vi "cm2nm_modify_spot_info.vi"(6 "Is Fiducial":bool, 8 "TransformedPt":bool, 9 "ArrayOfSpotNames":string[](array[string]), 10 "Current Session Information":T1={"CollectionOfPoints"=[{"MetaDataFile"=path "/INL Macintosh/Users/timothymcjunkin/Desktop/Diffusion couple/MXRD 9-13-10/Fid1.UXD", "X"=-4782.0, "Y"=12990.0, "Group"=1, "Z"=350.3, "Rotation"=1.5707963267948966, "Fiducial"=TRUE, "Magnification"=0.0, "Working_Distance"=0.0, "Notes"="", "Location Name/ID"="F1", "OtherRelatedDataFiles"=[], "Available"=TRUE}, {"MetaDataFile"=path "/INL Macintosh/Users/timothymcjunkin/Desktop/Diffusion couple/MXRD 9-13-10/Fid3B.UXD", "X"=-12864.0, "Y"=-4936.0, "Group"=1, "Z"=512.5999999999999, "Rotation"=1.5707963267948966, "Fiducial"=TRUE, "Magnification"=0.0, "Working_Distance"=0.0, "Notes"="", "Location Name/ID"="F3B", "OtherRelatedDataFiles"=[], "Available"=FALSE}, {"MetaDataFile"=path "/INL Macintosh/Users/timothymcjunkin/Desktop/Diffusion couple/MXRD 9-13-10/Fid5C.UXD", "X"=4762.0, "Y"=-13159.0, "Group"=1, "Z"=512.5999999999999, "Rotation"=1.5707963267948966, "Fiducial"=TRUE, "Magnification"=0.0, "Working_Distance"=0.0, "Notes"="", "Location Name/ID"="F5C", "OtherRelatedDataFiles"=[], "Available"=TRUE}, {"MetaDataFile"=path "", "X"=162.40381449303823, "Y"=-31.01324453854977, "Group"=1, "Z"=430.4482310236498, "Rotation"=0.0, "Fiducial"=FALSE, "Magnification"=0.0, "Working_Distance"=0.0, "Notes"="", "Location Name/ID"="Interface_corrected", "OtherRelatedDataFiles"=[], "Available"=FALSE}, {"MetaDataFile"=path "/INL Macintosh/Users/timothymcjunkin/Desktop/Diffusion couple/MXRD 9-13-10/Center.UXD", "X"=163.0, "Y"=44.0, "Group"=1, "Z"=-192.39999999999998, "Rotation"=-0.8089757988093471, "Fiducial"=FALSE, "Magnification"=0.0, "Working_Distance"=0.0, "Notes"="", "Location Name/ID"="interface_Manual_find", "OtherRelatedDataFiles"=[], "Available"=FALSE}, {"MetaDataFile"=path "", "X"=1407.972144786283, "Y"=-1304.0831828104674, "Group"=1, "Z"=435.6245662356068, "Rotation"=0.0, "Fiducial"=FALSE, "Magnification"=0.0, "Working_Distance"=0.0, "Notes"="", "Location Name/ID"="Corner_correcte_S1", "OtherRelatedDataFiles"=[], "Available"=FALSE}, {"MetaDataFile"=path "/INL Macintosh/Users/timothymcjunkin/Desktop/Diffusion couple/MXRD 9-13-10/Corner.UXD", "X"=1397.752237926863, "Y"=-1316.5905644166705, "Group"=1, "Z"=435.75379333055236, "Rotation"=-0.6331076967321386, "Fiducial"=FALSE, "Magnification"=0.0, "Working_Distance"=0.0, "Notes"="", "Location Name/ID"="Corner_correcte_S1_fix", "OtherRelatedDataFiles"=[], "Available"=FALSE}], "Instrument"=3, "CollectionFile"=path "/INL Macintosh/Users/timothymcjunkin/Desktop/Diffusion couple/MXRD 9-13-10/xrd_session_for_corrected.xml", "Session Name/ID"="xrd_test", "SessionNotes"="Sample moved to XRD"} {"Instrument" items=["Unknown", "Phillips SEM IRC", "JEOL 7000F EML_MFC", "MXRD MFC", "JEOL_EPMA"]; "CollectionOfPoints"."Rotation" min=-37480660.29033894 max=37480660.27288565}, 11 "Input of Spot information":T2={"MetaDataFile"=path "/INL Macintosh/Users/timothymcjunkin/Desktop/Diffusion couple/MXRD 9-13-10/Corner.UXD", "X"=1346.0, "Y"=-1254.0, "Group"=0, "Z"=-87.9, "Rotation"=-0.6331076967321386, "Fiducial"=FALSE, "Magnification"=0.0, "Working_Distance"=0.0, "Notes"="", "Location Name/ID"="", "OtherRelatedDataFiles"=[], "Available"=FALSE} {"Rotation" min=-37480660.29033894 max=37480660.27288565}) -> (0 "Output of Spot information":T2={"MetaDataFile"=path "/INL Macintosh/Users/timothymcjunkin/Desktop/Diffusion couple/MXRD 9-13-10/Corner.UXD", "X"=1346.0, "Y"=-1254.0, "Group"=0, "Z"=-87.9, "Rotation"=-0.6331076967321386, "Fiducial"=FALSE, "Magnification"=0.0, "Working_Distance"=0.0, "Notes"="", "Location Name/ID"="", "OtherRelatedDataFiles"=[], "Available"=FALSE} {"Rotation" min=-37480660.29033894 max=37480660.27288565}, 1 "Current Session Information Out":T1={"CollectionOfPoints"=[{"MetaDataFile"=path "/INL Macintosh/Users/timothymcjunkin/Desktop/Diffusion couple/MXRD 9-13-10/Fid1.UXD", "X"=-4782.0, "Y"=12990.0, "Group"=1, "Z"=350.3, "Rotation"=1.5707963267948966, "Fiducial"=TRUE, "Magnification"=0.0, "Working_Distance"=0.0, "Notes"="", "Location Name/ID"="F1", "OtherRelatedDataFiles"=[], "Available"=TRUE}, {"MetaDataFile"=path "/INL Macintosh/Users/timothymcjunkin/Desktop/Diffusion couple/MXRD 9-13-10/Fid3B.UXD", "X"=-12864.0, "Y"=-4936.0, "Group"=1, "Z"=512.5999999999999, "Rotation"=1.5707963267948966, "Fiducial"=TRUE, "Magnification"=0.0, "Working_Distance"=0.0, "Notes"="", "Location Name/ID"="F3B", "OtherRelatedDataFiles"=[], "Available"=FALSE}, {"MetaDataFile"=path "/INL Macintosh/Users/timothymcjunkin/Desktop/Diffusion couple/MXRD 9-13-10/Fid5C.UXD", "X"=4762.0, "Y"=-13159.0, "Group"=1, "Z"=512.5999999999999, "Rotation"=1.5707963267948966, "Fiducial"=TRUE, "Magnification"=0.0, "Working_Distance"=0.0, "Notes"="", "Location Name/ID"="F5C", "OtherRelatedDataFiles"=[], "Available"=TRUE}, {"MetaDataFile"=path "", "X"=162.40381449303823, "Y"=-31.01324453854977, "Group"=1, "Z"=430.4482310236498, "Rotation"=0.0, "Fiducial"=FALSE, "Magnification"=0.0, "Working_Distance"=0.0, "Notes"="", "Location Name/ID"="Interface_corrected", "OtherRelatedDataFiles"=[], "Available"=FALSE}, {"MetaDataFile"=path "/INL Macintosh/Users/timothymcjunkin/Desktop/Diffusion couple/MXRD 9-13-10/Center.UXD", "X"=163.0, "Y"=44.0, "Group"=1, "Z"=-192.39999999999998, "Rotation"=-0.8089757988093471, "Fiducial"=FALSE, "Magnification"=0.0, "Working_Distance"=0.0, "Notes"="", "Location Name/ID"="interface_Manual_find", "OtherRelatedDataFiles"=[], "Available"=FALSE}, {"MetaDataFile"=path "", "X"=1407.972144786283, "Y"=-1304.0831828104674, "Group"=1, "Z"=435.6245662356068, "Rotation"=0.0, "Fiducial"=FALSE, "Magnification"=0.0, "Working_Distance"=0.0, "Notes"="", "Location Name/ID"="Corner_correcte_S1", "OtherRelatedDataFiles"=[], "Available"=FALSE}, {"MetaDataFile"=path "/INL Macintosh/Users/timothymcjunkin/Desktop/Diffusion couple/MXRD 9-13-10/Corner.UXD", "X"=1397.752237926863, "Y"=-1316.5905644166705, "Group"=1, "Z"=435.75379333055236, "Rotation"=-0.6331076967321386, "Fiducial"=FALSE, "Magnification"=0.0, "Working_Distance"=0.0, "Notes"="", "Location Name/ID"="Corner_correcte_S1_fix", "OtherRelatedDataFiles"=[], "Available"=FALSE}], "Instrument"=3, "CollectionFile"=path "/INL Macintosh/Users/timothymcjunkin/Desktop/Diffusion couple/MXRD 9-13-10/xrd_session_for_corrected.xml", "Session Name/ID"="xrd_test", "SessionNotes"="Sample moved to XRD"} {"Instrument" items=["Unknown", "Phillips SEM IRC", "JEOL 7000F EML_MFC", "MXRD MFC", "JEOL_EPMA"]; "CollectionOfPoints"."Rotation" min=-37480660.29033894 max=37480660.27288565}, 3 "Cancel":bool)   [LabVIEW 2010]
uses:
  cm2nm_coordinate_information_v2.ctl
  cm2nm_sample_set.ctl
panel:
  in  "Group Coding":i32
  in  "Boolean 2":bool
  in  "Boolean":bool
  out "MetaDataAvailable":bool caption="Is a Fiducial"
  out "error out":errorcluster
  in  "Is a Fiducial":bool
  in  "Notes:":string
  in  "Tab Control":T3(tab)
  in  "Tilt":dbl
  in  "Stage Rotation":dbl
  in  "Get Coordinates from Meta File":bool
  in  "Press to Move to Next\nInformation Screen":bool
  in  "Spot Name":string
  in  "Z-Position":dbl
  in  "Y-Position":dbl
  in  "X-Position":dbl
  in  "MetaDataFile":path
  in  "Cancel2":bool caption="Cancel Adding \nthis Point to \nthe DataBase"
  in  "Add A Spot Related Data File":bool caption="Add Another File\nRelated to this Spot"
  in  "Goto Previous Screen":bool caption="Press to Move to \nPrevious Screen"
  in  "Press to goto final Screen":bool caption="Press to Move to Next\nInformation Screen"
  out "OtherRelatedDataFiles":T4(array[cluster])
  in  "Cancel3":bool caption="Cancel Adding \nthis Point to \nthe DataBase"
  in  "Go Back to Correct":bool caption="Some information\nis Incorrect or \nWrong"
  in  "Cancel":bool caption="Cancel Adding \nthis Point to \nthe DataBase"
  in  "AddToDataBase":bool caption="Information is\nCorrect Add the\nPoint"
  # "Enter or confirm the\nspot  name and positions\n\nIf Metafile is available \nselect it in the MetaDatafile\nField and click Use MetaFile\nto extract MetaData\nFrom the file."
  # "This form allows you\nto add any number of\nfiles related to this\nspot on the sample.\nFor example spectra\nfiles or images other\nthan the file \ncontaining meta data."
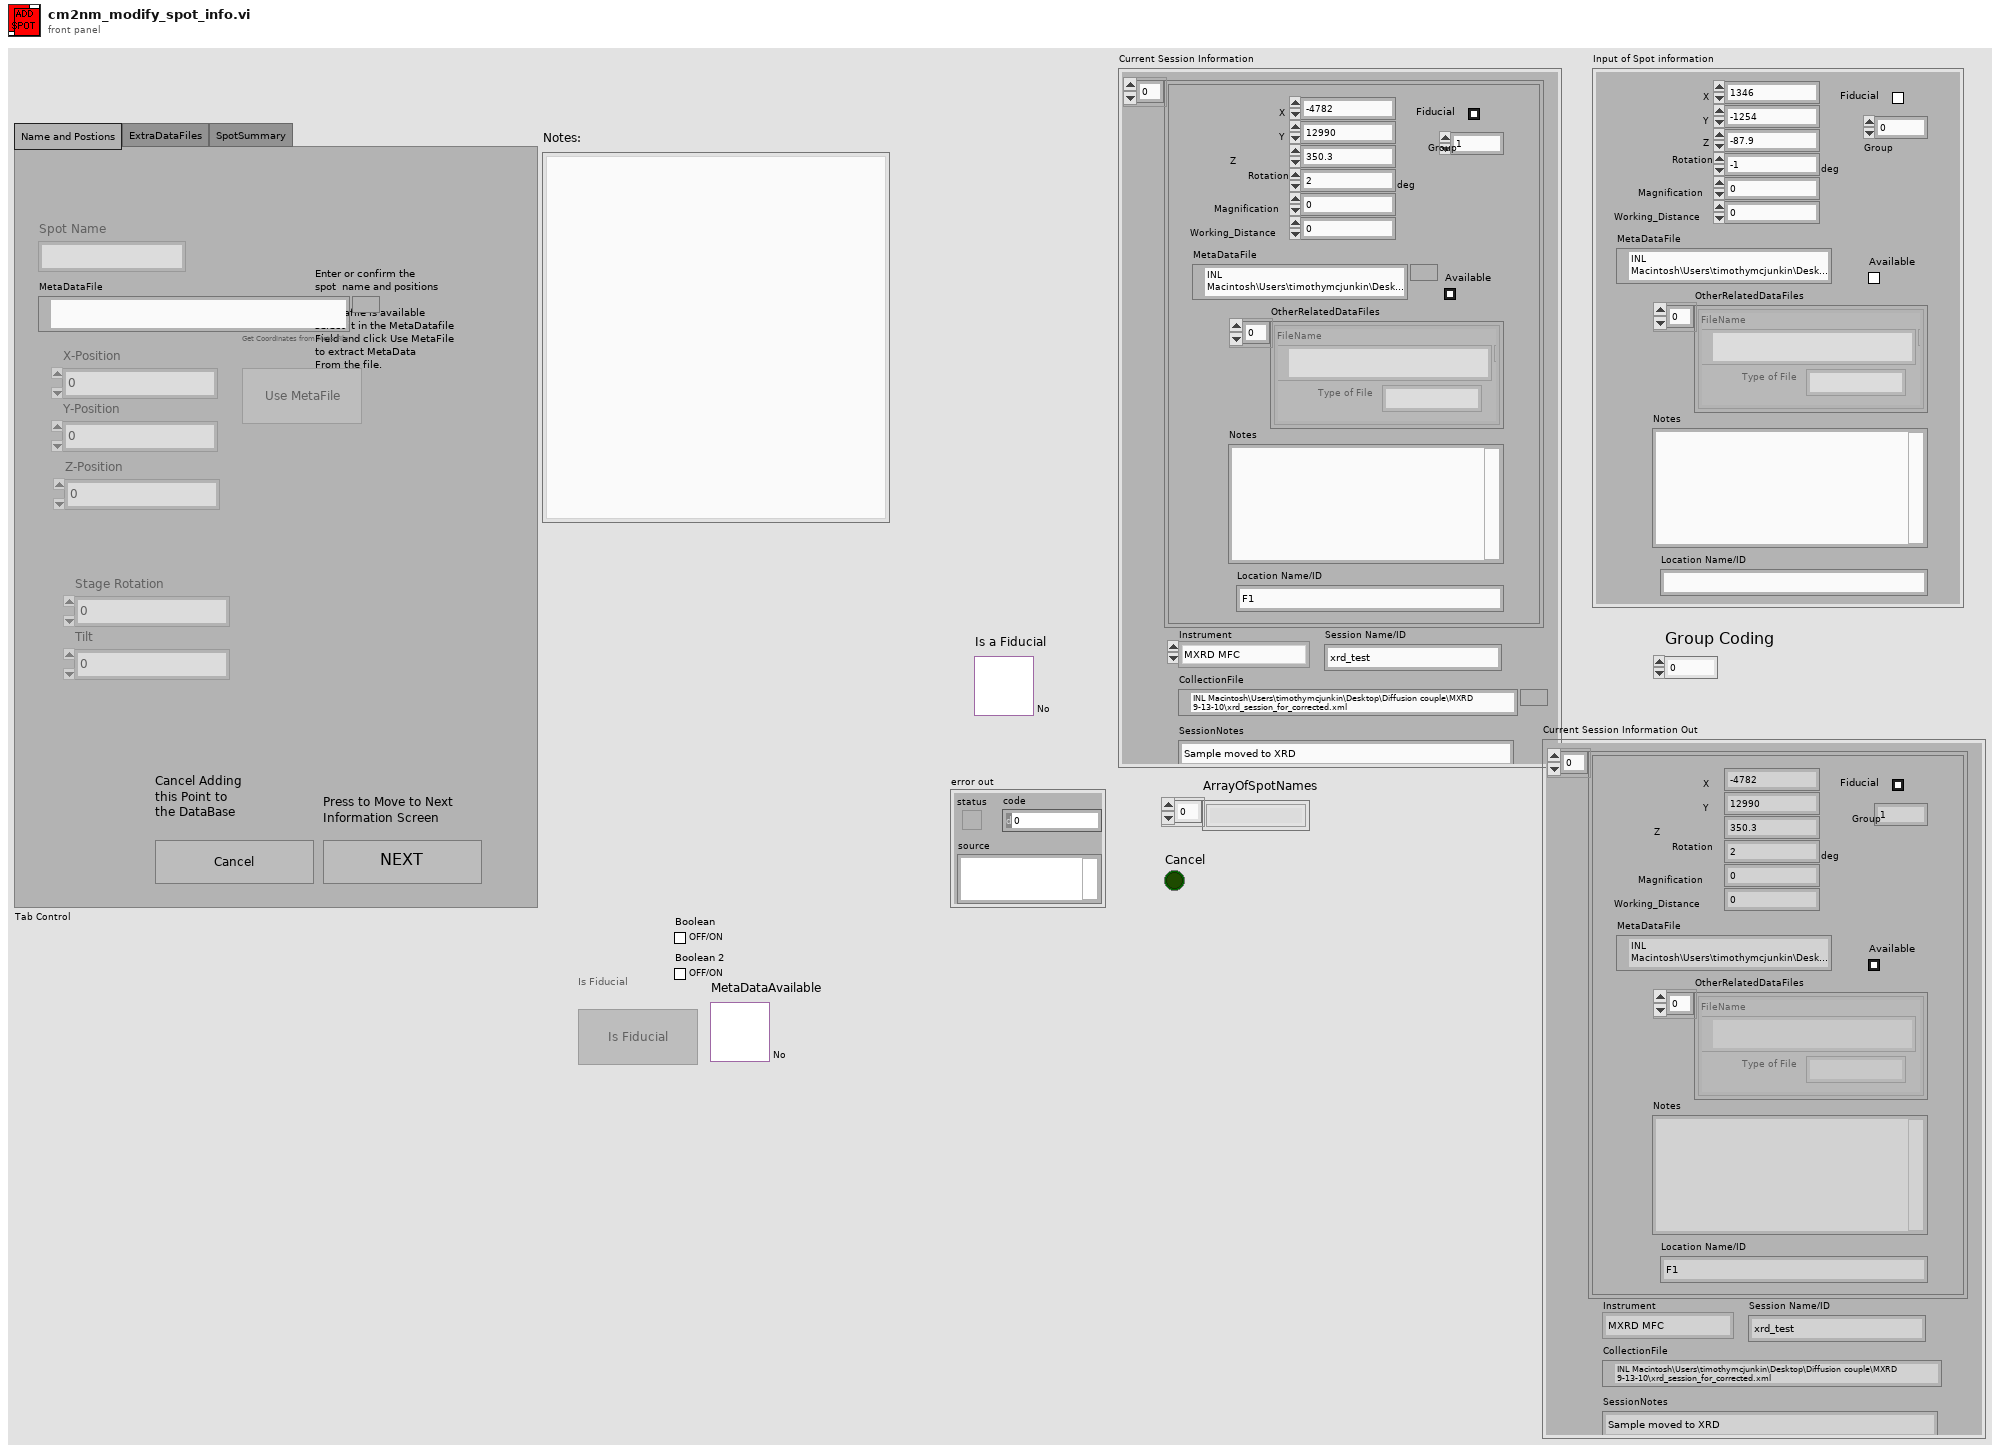
[diagram p1: front panel]
types:
  T1 = typedef "cm2nm_sample_set.ctl" = cluster{"CollectionOfPoints":T2[], "Instrument":u16, "CollectionFile":path, "Session Name/ID":string, "SessionNotes":string}
  T2 = typedef "cm2nm_coordinate_information_v2.ctl" = cluster{"MetaDataFile":path, "X":dbl, "Y":dbl, "Group":i32, "Z":dbl, "Rotation":dbl[unit], "Fiducial":bool, "Magnification":dbl, "Working_Distance":dbl, "Notes":string, "Location Name/ID":string, "OtherRelatedDataFiles":cluster{"Type of File":string, "FileName":path}[], "Available":bool}
  T3 = enum32{"Name and Postions", "ExtraDataFiles", "SpotSummary"}
  T4 = cluster{"Type of File":string, "FileName":path}[]
  T5 = enum32{"Name and Postions", "ExtraDataFiles", "SpotSummary", "Inputs"}
  T6 = enum8{"Enabled", "Disabled", "Disabled and Grayed Out"}
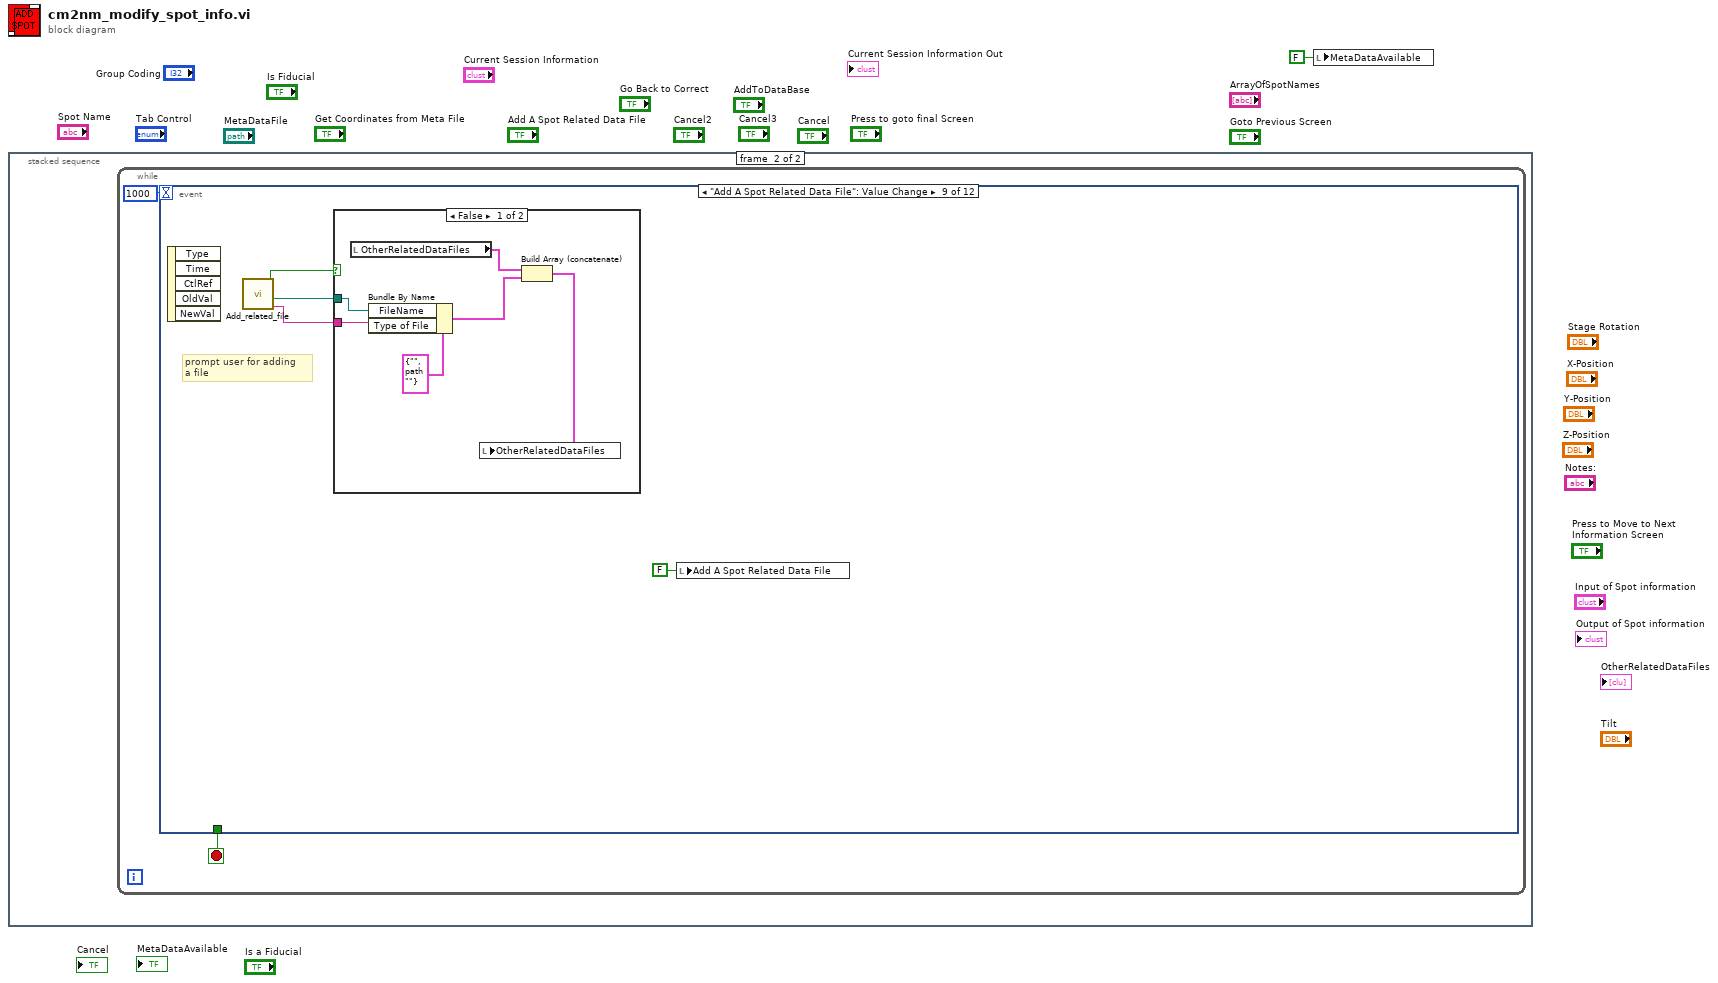
[diagram p0: block diagram]
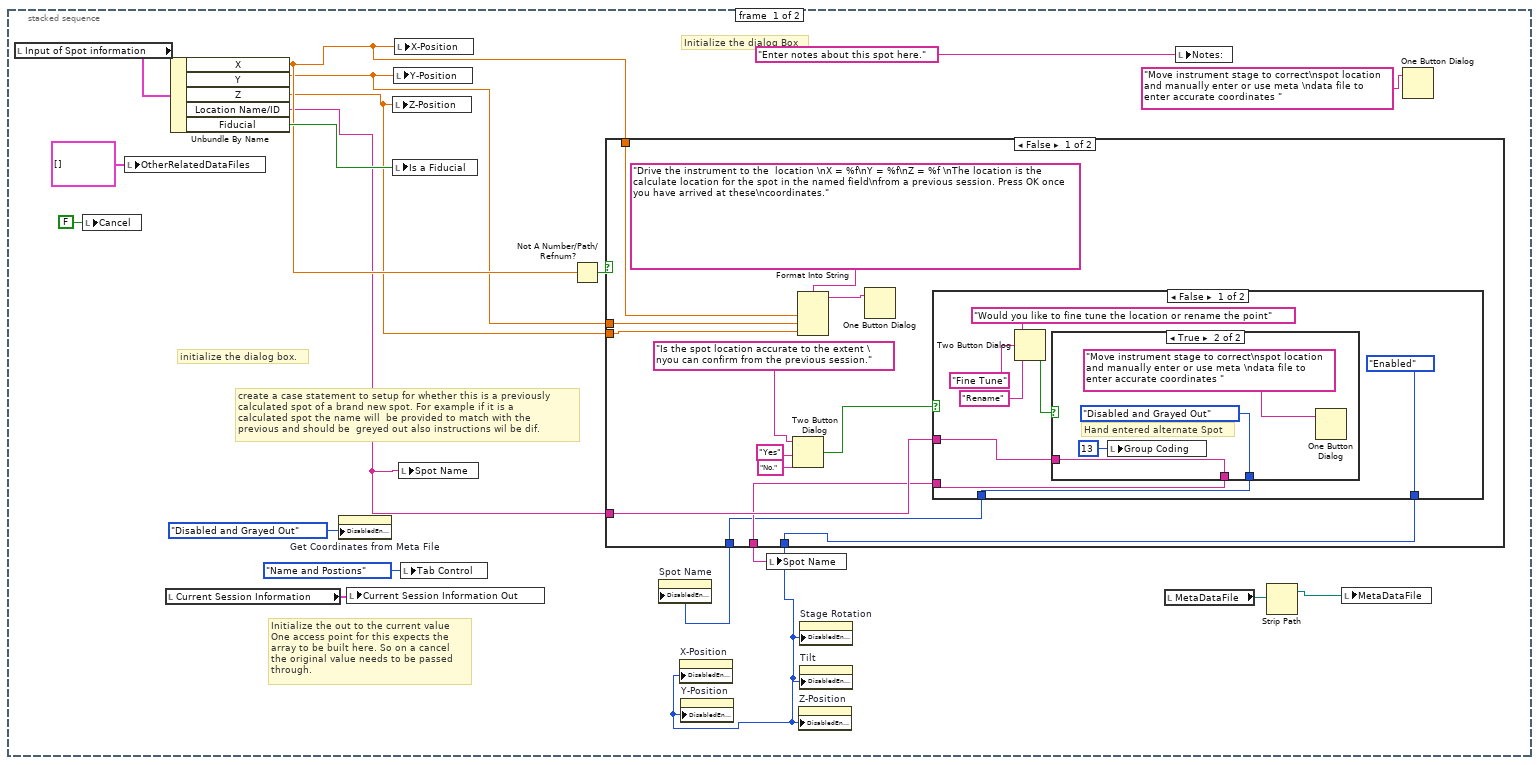
[diagram p2: hidden frame]
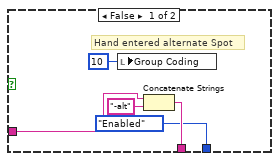
[diagram p3: hidden frame]
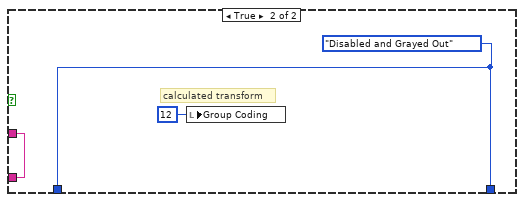
[diagram p4: hidden frame]
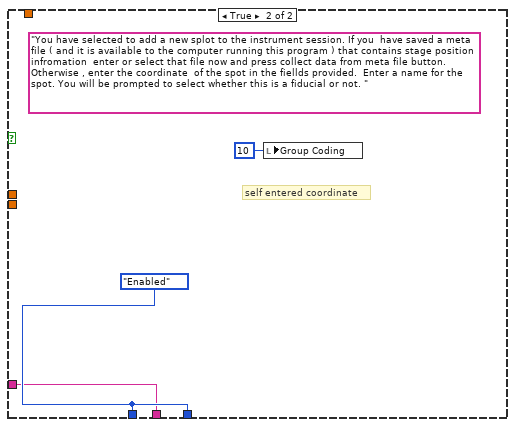
[diagram p5: hidden frame]
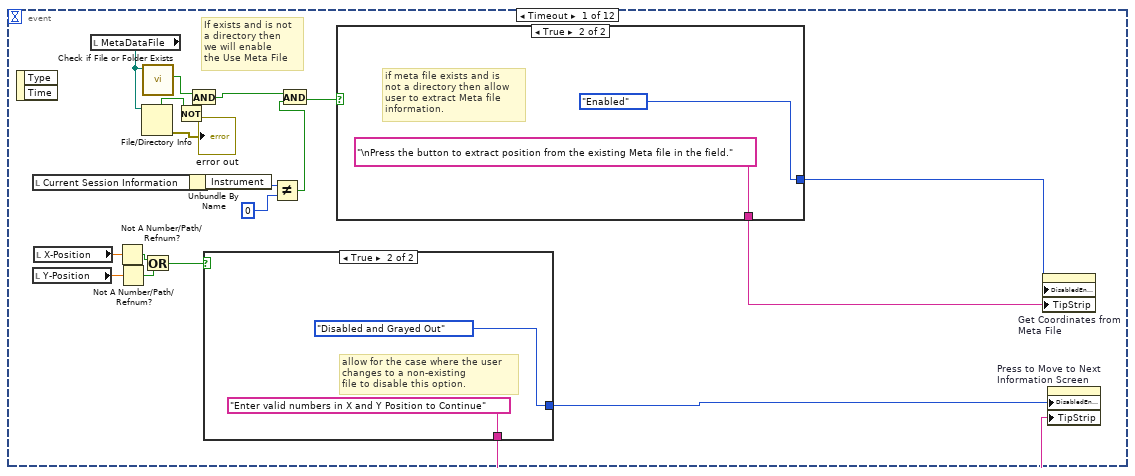
[diagram p6: hidden frame]
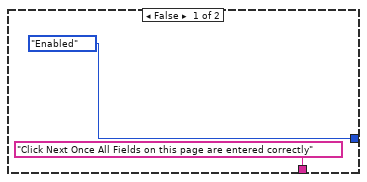
[diagram p7: hidden frame]
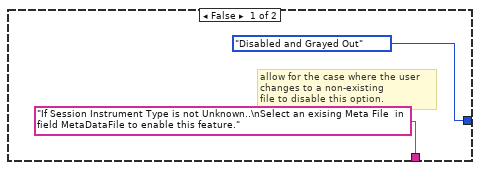
[diagram p8: hidden frame]
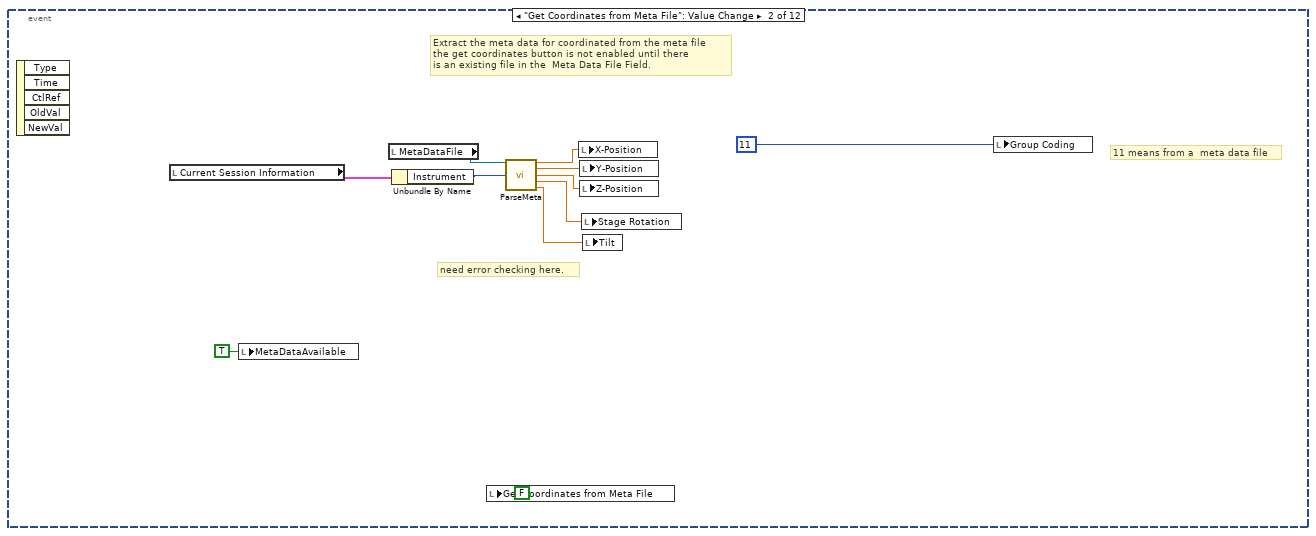
[diagram p9: hidden frame]
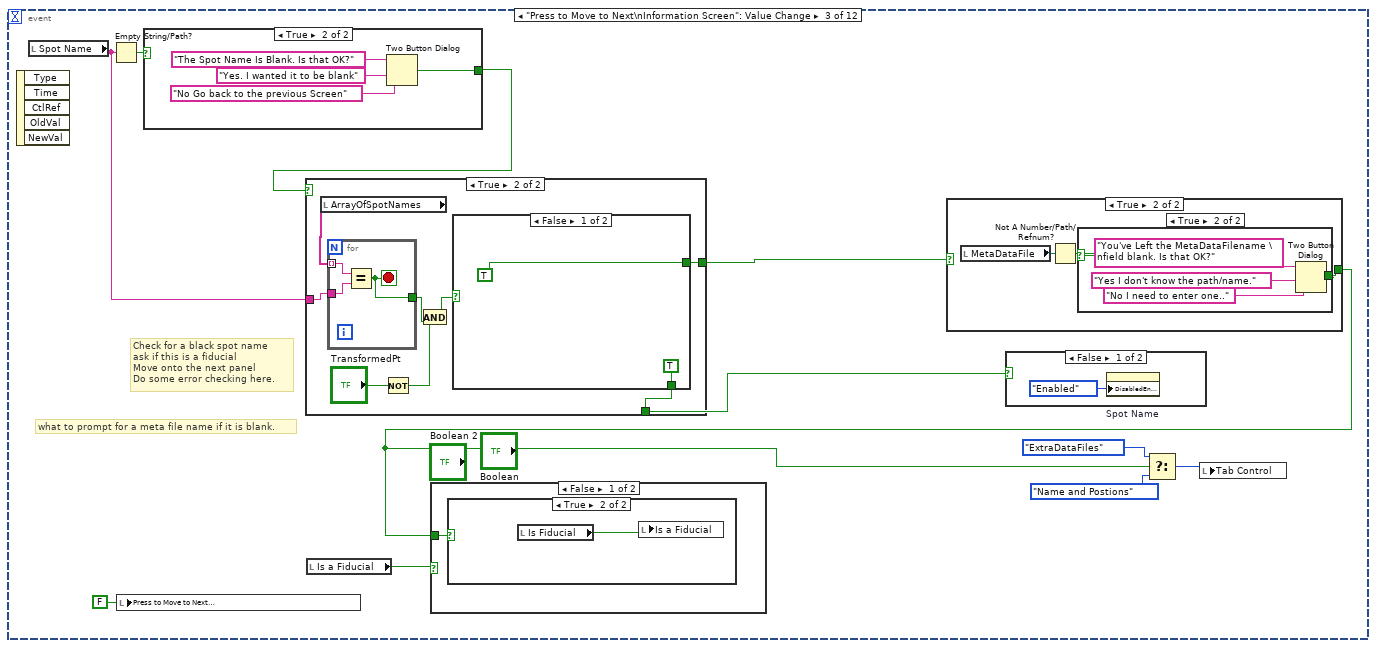
[diagram p10: hidden frame]
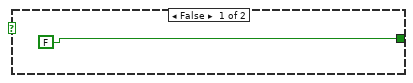
[diagram p14: hidden frame]
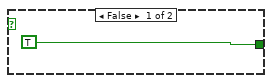
[diagram p15: hidden frame]
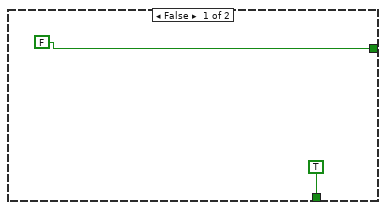
[diagram p16: hidden frame]
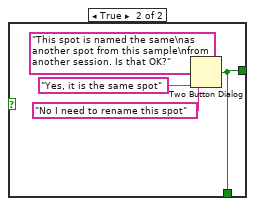
[diagram p17: hidden frame]
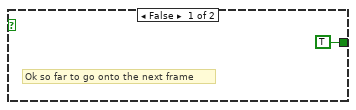
[diagram p18: hidden frame]
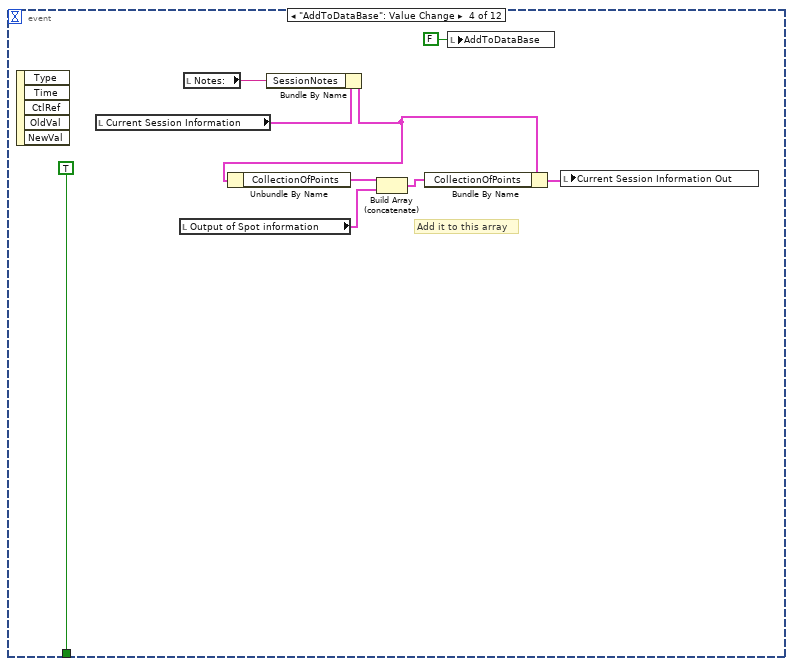
[diagram p19: hidden frame]
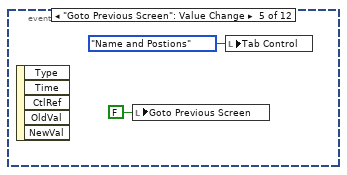
[diagram p20: hidden frame]
diagram:
  n1 = stacked-sequence {
    frame #0 {
      # "Initialize the out to the current value\nOne access point for this expects the\narray to be built here. So on a cancel\nthe original value needs to be passed\nthrough."
      # "Initialize the dialog Box"
      # "create a case statement to setup for whether this is a previously\ncalculated spot of a brand new spot. For example if it is a\ncalculated spot the name will  be provided to match with the \nprevious and should be  greyed out also instructions wil be dif."
      # "initialize the dialog box."
      n2 = local read "Input of Spot information"() -> (w20:T2)
      n3 = local write "Cancel"(FALSE ("Cancel")) -> ()
      n4 = local write "OtherRelatedDataFiles"(T4 [] ("OtherRelatedDataFiles")) -> ()
      n5 = local read "Current Session Information"() -> (w8:T1)
      n6 = Unbundle By Name(w20) -> ("X"=w16:dbl, "Y"=w15:dbl, "Z"=w3:dbl, "Location Name/ID"=w6:string, "Fiducial"=w19:bool)
      n7 = property on="Get Coordinates from Meta File" class="Bool (strict)"("DisabledEnum"=T6."Disabled and Grayed Out" ("Disabled")) -> ()  [unwired: 2 in, 2 out]
      n8 = local write "Current Session Information Out"(w8) -> ()
      n9 = local write "Z-Position"(w3) -> ()
      n10 = local write "Is a Fiducial"(w19) -> ()
      n11 = local write "Y-Position"(w15) -> ()
      n12 = local write "X-Position"(w16) -> ()
      n13 = local write "Spot Name"(w6) -> ()
      n14 = local write "Tab Control"(T5."Name and Postions" ("Tab Control")) -> ()
      n15 = Not A Number/Path/Refnum?(number/path/refnum=w16) -> (NaN/Path/Refnum?=w18:bool)
      n16 = case shown="False" w18 {
        tunnel: [w24 w56] -> w14
        tunnel: w16 -> [w32 _]
        tunnel: w15 -> [w31 _]
        tunnel: [w21 w56] -> w13
        tunnel: w6 -> [w23 w55]
        tunnel: [w22 w55] -> w12
        tunnel: w3 -> [w26 _]
        frame False {
          n17 = Two Button Dialog(message="Is the spot location accurate to the extent \nyou can confirm from the previous session.", 1:"No." ("F button name (\"Cancel\")"), 2:"Yes" ("T button name (\"OK\")")) -> (T button?=w25:bool)
          n18 = Format Into String(format string="Drive the instrument to the  location \nX = %f\nY = %f\nZ = %f \nThe location is the calculate location for the spot in the named field\nfrom a previous session. Press OK once you have arrived at these\ncoordinates.", w32, w31, w26) -> (resulting string=w30:string)  [unwired: 2 in, 1 out]
          n19 = One Button Dialog ("Drive to the Calculated Coordinates")(message=w30) -> ()  [unwired: 1 in, 1 out]
          n20 = case shown="False" w25 {
            tunnel: [T6."Enabled" ("Disabled") w52] -> w24
            tunnel: w23 -> [w36 w53]
            tunnel: [w35 w53] -> w22
            tunnel: [w34 w52] -> w21
            frame False {
              n21 = Two Button Dialog(message="Would you like to fine tune the location or rename the point", 1:"Rename" ("F button name (\"Cancel\")"), 2:"Fine Tune" ("T button name (\"OK\")")) -> (T button?=w37:bool)
              n22 = case shown="True" w37 {
                tunnel: w36 -> [w45 w50]
                tunnel: [w44 w50] -> w35
                tunnel: [T6."Enabled" ("Disabled") T6."Disabled and Grayed Out" ("Disabled")] -> w34
                frame False {
                  # "Hand entered alternate Spot"
                  n23 = local write "Group Coding"(10 ("Group Coding")) -> ()
                  n24 = Concatenate Strings(w45, "-alt" ("string")) -> (w44:string)
                }
                frame True {
                  # "Hand entered alternate Spot"
                  n25 = local write "Group Coding"(13 ("Group Coding")) -> ()
                  n26 = One Button Dialog ("Drive to the Calculated Coordinates")(message="Move instrument stage to correct\nspot location and manually enter or use meta \ndata file to enter accurate coordinates ") -> ()  [unwired: 1 in, 1 out]
                }
              }
            }
            frame True {
              w52 = T6."Disabled and Grayed Out" ("Disabled")
              # "calculated transform"
              n27 = local write "Group Coding"(12 ("Group Coding")) -> ()
            }
          }
        }
        frame True {
          w56 = T6."Enabled" ("Disabled")
          (unwired) "You have selected to add a new splot to the instrument session. If you  have saved a meta file ( and it is available to the computer running this program ) that contains stage position infromation  enter or select that file now and press collect data from meta file button. Otherwise , enter the coordinate  of the spot in the fiellds provided.  Enter a name for the spot. You will be prompted to select whether this is a fiducial or not. "
          # "self entered coordinate"
          n28 = local write "Group Coding"(10 ("Group Coding")) -> ()
        }
      }
      n29 = property on="Spot Name" class="Str"("DisabledEnum"=w13) -> ()  [unwired: 2 in, 2 out]
      n30 = property on="X-Position" class="DigNum (strict)"("DisabledEnum"=w14) -> ()  [unwired: 2 in, 2 out]
      n31 = property on="Y-Position" class="DigNum (strict)"("DisabledEnum"=w14) -> ()  [unwired: 2 in, 2 out]
      n32 = local write "Spot Name"(w12) -> ()
      n33 = property on="Z-Position" class="DigNum (strict)"("DisabledEnum"=w14) -> ()  [unwired: 2 in, 2 out]
      n34 = property on="Stage Rotation" class="DigNum (strict)"("DisabledEnum"=w14) -> ()  [unwired: 2 in, 2 out]
      n35 = property on="Tilt" class="DigNum (strict)"("DisabledEnum"=w14) -> ()  [unwired: 2 in, 2 out]
      n36 = local read "MetaDataFile"() -> (w5:path)
      n37 = local write "Notes:"("Enter notes about this spot here." ("Notes:")) -> ()
      n38 = Strip Path(path=w5) -> (stripped path=w4:path)  [unwired: 1 out]
      n39 = local write "MetaDataFile"(w4) -> ()
      n40 = One Button Dialog ("Drive to the Calculated Coordinates")(message="Move instrument stage to correct\nspot location and manually enter or use meta \ndata file to enter accurate coordinates ") -> ()  [unwired: 1 in, 1 out]
    }
    frame #1 {
      n41 = while {
        stop <- w57 stop-if-true
        n42 = event shown="[8] \"Add A Spot Related Data File\": Value Change" {
          selector: _ -> [_ _ _ _ _ _ _ _ _ _ _ _]
          dyn-events: _ -> [_ _ _ _ _ _ _ _ _ _ _ _]
          timeout: 1000 -> [_ _ _ _ _ _ _ _ _ _ _ _]
          tunnel: [_ _ _ TRUE ("T button?") _ _ _ w188 _ _ _ _] -> w57
          event Timeout {
            # "If exists and is not\na directory then\nwe will enable \nthe Use Meta File"
            n43 = event-data() -> ()  [unwired: 1 in, 2 out]
            n44 = local read "Current Session Information"() -> (w63:T1)
            n45 = local read "Y-Position"() -> (w67:dbl)
            n46 = local read "X-Position"() -> (w68:dbl)
            n47 = local read "MetaDataFile"() -> (w71:path)
            n48 = Not A Number/Path/Refnum?(number/path/refnum=w68) -> (NaN/Path/Refnum?=w66:bool)
            n49 = Not A Number/Path/Refnum?(number/path/refnum=w67) -> (NaN/Path/Refnum?=w65:bool)
            n50 = File/Directory Info(path=w71) -> (directory=w78:bool, error out=→"error out":errorcluster)  [unwired: 1 in, 5 out]
            n51 = call <vilib>:"Check if File or Folder Exists.vi"("path"=w71) -> ("file or folder exists?"=w76:bool)  [unwired: 8 in, 2 out]
            n52 = Or(x=w66, y=w65) -> (x .or. y?=w64:bool)
            n53 = Not(x=w78) -> (.not. x?=w77:bool)
            n54 = And(x=w76, y=w77) -> (x .and. y?=w72:bool)
            n55 = Unbundle By Name(w63) -> ("Instrument"=w62:u16)
            n56 = case shown="True" w64 {
              tunnel: [T6."Enabled" ("Disabled") T6."Disabled and Grayed Out" ("Disabled")] -> w70
              tunnel: ["Click Next Once All Fields on this page are entered correctly" ("Tip Strip") "Enter valid numbers in X and Y Position to Continue" ("Tip Strip")] -> w69
              frame False {
              }
              frame True {
                # "allow for the case where the user\nchanges to a non-existing\nfile to disable this option."
              }
            }
            n57 = Not Equal?(x=w62, y=u16 0) -> (x != y?=w59:bool)
            n58 = And(x=w72, y=w59) -> (x .and. y?=w60:bool)
            n59 = case shown="True" w60 {
              tunnel: [T6."Disabled and Grayed Out" ("Disabled") T6."Enabled" ("Disabled")] -> w74
              tunnel: ["If Session Instrument Type is not Unknown..\nSelect an exising Meta File  in field MetaDataFile to enable this feature." ("Tip Strip") "\nPress the button to extract position from the existing Meta file in the field." ("Tip Strip")] -> w73
              frame False {
                # "allow for the case where the user\nchanges to a non-existing\nfile to disable this option."
              }
              frame True {
                # "if meta file exists and is\nnot a directory then allow \nuser to extract Meta file \ninformation."
              }
            }
            n60 = property on="Get Coordinates from Meta File" class="Bool (strict)"("DisabledEnum"=w74, "TipStrip"=w73) -> ()  [unwired: 2 in, 2 out]
            n61 = property on="Press to Move to Next\nInformation Screen" class="Bool (strict)"("DisabledEnum"=w70, "TipStrip"=w69) -> ()  [unwired: 2 in, 2 out]
          }
          event "Get Coordinates from Meta File": Value Change {
            # "11 means from a  meta data file"
            # "need error checking here."
            # "Extract the meta data for coordinated from the meta file\nthe get coordinates button is not enabled until there\nis an existing file in the  Meta Data File Field."
            n62 = event-data() -> ()  [unwired: 1 in, 5 out]
            n63 = local read "Current Session Information"() -> (w88:T1)
            n64 = local write "MetaDataAvailable"(TRUE ("MetaDataAvailable")) -> ()
            n65 = local read "MetaDataFile"() -> (w96:path)
            n66 = Unbundle By Name(w88) -> ("Instrument"=w95:u16)
            n67 = local write "Get Coordinates from Meta File"(FALSE ("Get Coords")) -> ()
            n68 = call "ParseMeta.vi"("Path"=w96, "Instrument"=w95) -> ("X-stage (um)"=w94:dbl, "Y-stage (um)"=w93:dbl, "Z-stage (um)"=w92:dbl, "R-stage (deg)"=w91:dbl, "StageTilt"=w90:dbl)  [unwired: 1 in, 8 out]
            n69 = local write "X-Position"(w94) -> ()
            n70 = local write "Y-Position"(w93) -> ()
            n71 = local write "Z-Position"(w92) -> ()
            n72 = local write "Stage Rotation"(w91) -> ()
            n73 = local write "Tilt"(w90) -> ()
            n74 = local write "Group Coding"(11 ("Group Coding")) -> ()
          }
          event "Press to Move to Next\nInformation Screen": Value Change {
            # "what to prompt for a meta file name if it is blank."
            # "Check for a black spot name\nask if this is a fiducial\nMove onto the next panel\nDo some error checking here."
            n75 = event-data() -> ()  [unwired: 1 in, 5 out]
            n76 = local read "Spot Name"() -> (w105:string)
            n77 = Empty String/Path?(string/path=w105) -> (empty?=w107:bool)
            n78 = local write "Press to Move to Next\nInformation Screen"(FALSE ("Press to Move to Next\nInformation Screen")) -> ()
            n79 = case shown="True" w107 {
              tunnel: [TRUE ("T button?") w141] -> w106
              frame False {
                # "Ok so far to go onto the next frame"
              }
              frame True {
                n80 = Two Button Dialog(message="The Spot Name Is Blank. Is that OK?", 1:"No Go back to the previous Screen" ("F button name (\"Cancel\")"), 2:"Yes. I wanted it to be blank" ("T button name (\"OK\")")) -> (T button?=w141:bool)
              }
            }
            n81 = case shown="True" w106 {
              tunnel: w105 -> [_ w129]
              tunnel: [FALSE ("T button?") w127] -> w104
              tunnel: [TRUE ("T button?") w126] -> w99
              frame False {
              }
              frame True {
                n82 = local read "ArrayOfSpotNames"() -> (w130:string[])
                n83 = for {
                  tunnel: w130 -> [w139] mode=indexing
                  tunnel: w129 -> [w138]
                  tunnel: [w137] -> w128
                  stop <- w137 stop-if-true
                  n84 = Equal?(x=w139, y=w138) -> (x = y?=w137:bool)
                }
                n85 = Not(x="TransformedPt") -> (.not. x?=w123:bool)
                n86 = And(x=w123, y=w128) -> (x .and. y?=w125:bool)
                n87 = case shown="False" w125 {
                  tunnel: [TRUE ("T button?") w133] -> w127
                  tunnel: [TRUE ("T button?") w133] -> w126
                  frame False {
                  }
                  frame True {
                    n88 = Two Button Dialog(message="This spot is named the same\nas another spot from this sample\nfrom another session. Is that OK?", 1:"No I need to rename this spot" ("F button name (\"Cancel\")"), 2:"Yes, it is the same spot" ("T button name (\"OK\")")) -> (T button?=w133:bool)
                  }
                }
              }
            }
            n89 = local read "Is a Fiducial"() -> (w98:bool)
            n90 = case shown="True" w104 {
              tunnel: [FALSE ("T button?") w113] -> w100
              frame False {
              }
              frame True {
                n91 = local read "MetaDataFile"() -> (w115:path)
                n92 = Not A Number/Path/Refnum?(number/path/refnum=w115) -> (NaN/Path/Refnum?=w114:bool)
                n93 = case shown="True" w114 {
                  tunnel: [TRUE ("T button?") w117] -> w113
                  frame False {
                  }
                  frame True {
                    n94 = Two Button Dialog(message="You've Left the MetaDataFilename \nfield blank. Is that OK?", 1:"No I need to enter one.." ("F button name (\"Cancel\")"), 2:"Yes I don't know the path/name." ("T button name (\"OK\")")) -> (T button?=w117:bool)
                  }
                }
              }
            }
            n95 = case shown="False" w98 {
              tunnel: w100 -> [w109 _]
              frame False {
                n96 = case shown="True" w109 {
                  frame False {
                  }
                  frame True {
                    n97 = local read "Is Fiducial"() -> (w110:bool)
                    n98 = local write "Is a Fiducial"(w110) -> ()
                  }
                }
              }
              frame True {
              }
            }
            n99 = case shown="False" w99 {
              frame False {
                n100 = property on="Spot Name" class="Str"("DisabledEnum"=T6."Enabled" ("Disabled")) -> ()  [unwired: 2 in, 2 out]
              }
              frame True {
              }
            }
            n101 = Select(t=T5."ExtraDataFiles" ("Tab Control"), s=w100, f=T5."Name and Postions" ("Tab Control")) -> (s? t:f=w103:T5)
            n102 = local write "Tab Control"(w103) -> ()
          }
          event "AddToDataBase": Value Change {
            # "Add it to this array"
            n103 = event-data() -> ()  [unwired: 1 in, 5 out]
            n104 = local read "Current Session Information"() -> (w150:T1)
            n105 = local read "Output of Spot information"() -> (w148:T2)
            n106 = local read "Notes:"() -> (w145:string)
            n107 = Bundle By Name(cluster=w150, "SessionNotes"=w145) -> (w146:T1)
            n108 = Unbundle By Name(w146) -> ("CollectionOfPoints"=w149:T2[])
            n109 = Build Array (concatenate)(w149, w148) -> (w147:T2[])
            n110 = Bundle By Name(cluster=w146, "CollectionOfPoints"=w147) -> (w151:T1)
            n111 = local write "AddToDataBase"(FALSE ("AddToDataBase")) -> ()
            n112 = local write "Current Session Information Out"(w151) -> ()
          }
          event "Goto Previous Screen": Value Change {
            n113 = event-data() -> ()  [unwired: 1 in, 5 out]
            n114 = local write "Goto Previous Screen"(FALSE ("Goto Previous Screen")) -> ()
            n115 = local write "Tab Control"(T5."Name and Postions" ("Tab Control")) -> ()
          }
          event "X-Position", "Y-Position", "Z-Position", "MetaDataFile": Value Change {
            # "If user changes any of these from the interface then the values did not come\nfrom the meta file and the indicator should be false."
            n116 = event-data() -> ("CtlRef"=w156:refnum<vi>, "OldVal"=w158:variant, "NewVal"=w157:variant)  [unwired: 1 in, 2 out]
            n117 = local read "Group Coding"() -> (w159:i32)
            n118 = case shown="11" w159 {
              tunnel: w158 -> [_ _ w160]
              tunnel: w157 -> [_ _ _]
              tunnel: w156 -> [_ _ w161]
              frame 0, Default {
              }
              frame 10 {
                # "10 is ok  self entered no warning message for entering these values."
              }
              frame 11 {
                # "coding from meta data file"
                n119 = Two Button Dialog(message="You have modified values\nread from the meta data\nfile or the meta data file name\n. Do you want to do \nthis?  ", 1:"No revert to the old meta data Value" ("F button name (\"Cancel\")"), 2:"Yes, keep the new values" ("T button name (\"OK\")")) -> (T button?=w162:bool)
                n120 = case shown="False" w162 {
                  tunnel: w161 -> [w168 _]
                  tunnel: w160 -> [w166 _]
                  frame False {
                    n121 = property class="Ctl" props=["Value"](reference=w168) -> (reference out=w167:refnum<vi>)  [unwired: 1 in, 2 out]
                    n122 = property class="Ctl"(reference=w167, "Value"=w166) -> ()  [unwired: 1 in, 2 out]
                  }
                  frame True {
                    # "change to 10 so the user\ncan modify as needed"
                    n123 = local write "Group Coding"(10 ("Group Coding")) -> ()
                  }
                }
              }
            }
          }
          event "Spot Name": Value Change {
            n124 = event-data() -> ()  [unwired: 1 in, 5 out]
            n125 = local read "Spot Name"() -> (w170:string)
            n126 = local read "Current Session Information"() -> (w173:T1)
            n127 = Unbundle By Name(w173) -> ("CollectionOfPoints"=w172:T2[])
            n128 = for {
              tunnel: w172 -> [w186] mode=indexing
              tunnel: w170 -> [w184]
              tunnel: [w183] -> w171
              stop <- w183 stop-if-true
              n129 = Unbundle By Name(w186) -> ("Location Name/ID"=w185:string)
              n130 = Equal?(x=w184, y=w185) -> (x = y?=w183:bool)
            }
            n131 = case shown="True" w171 {
              tunnel: w170 -> [_ w179]
              frame False {
              }
              frame True {
                n132 = Random Number (0-1)() -> (number: 0 to 1=w182:dbl)
                n133 = Multiply(x=w182, y=10000) -> (x*y=w177:dbl)
                n134 = Round Toward -Infinity(1:w177) -> (0:w176:dbl)
                n135 = To Unsigned Long Integer(number=w176) -> (unsigned 32bit integer=w175:u32)
                n136 = Format Into String(w175) -> (resulting string=w178:string)  [unwired: 3 in, 1 out]
                n137 = Concatenate Strings(w179, w178) -> (w180:string)
                n138 = property on="Spot Name" class="Str"("Val(Sgnl)"=w180) -> ()  [unwired: 2 in, 2 out]
                n139 = One Button Dialog(message="You have chosen a spot name that duplicates one in this session. \nA random number has been appended to it.") -> ()  [unwired: 1 in, 1 out]
              }
            }
          }
          event "Cancel2", "Cancel3", "Cancel": Value Change {
            w187 = FALSE ("Cancel")
            n140 = event-data() -> ()  [unwired: 1 in, 5 out]
            n141 = Two Button Dialog(message="You have selected cancel adding this spot to the DataBase. Press \"Yes\" if that's what you intended.", 1:"Don't Cancel this Spot" ("F button name (\"Cancel\")"), 2:"YES. do not save this spot" ("T button name (\"OK\")")) -> (T button?=w188:bool)
            n142 = local write "Cancel2"(w187) -> ()
            n143 = local write "Cancel"(w187) -> ()
            n144 = local write "Cancel3"(w187) -> ()
            n145 = local write "Cancel"(w188) -> ()
          }
          event "Add A Spot Related Data File": Value Change {
            # "prompt user for adding\na file"
            n146 = event-data() -> ()  [unwired: 1 in, 5 out]
            n147 = call "Add_related_file.vi"() -> ("Type or Description of File Out"=w193:string, "Path_out"=w194:path, "Cancelled?"=w195:bool)  [unwired: 9 in]
            n148 = case shown="False" w195 {
              tunnel: w194 -> [w199 _]
              tunnel: w193 -> [w198 _]
              frame False {
                n149 = local read "OtherRelatedDataFiles"() -> (w201:T4)
                n150 = Bundle By Name(cluster=cluster{"Type of File":string, "FileName":path} {"Type of File"="", "FileName"=path ""} ("element"), "FileName"=w199, "Type of File"=w198) -> (w197:cluster{"Type of File":string, "FileName":path})
                n151 = Build Array (concatenate)(w201, w197) -> (w196:T4)
                n152 = local write "OtherRelatedDataFiles"(w196) -> ()
              }
              frame True {
              }
            }
            n153 = local write "Add A Spot Related Data File"(FALSE ("Add A Spot Related Data File")) -> ()
          }
          event "Press to goto final Screen": Value Change {
            w203 = 0.0 ("Magnification")
            # "new coding on group\n10 - is a user entered item"
            n154 = event-data() -> ()  [unwired: 1 in, 5 out]
            n155 = local read "Group Coding"() -> (w202:i32)
            n156 = local write "Tab Control"(T3."SpotSummary" ("Tab Control")) -> ()
            n157 = local read "Stage Rotation"() -> (w210:dbl)
            n158 = local read "Is a Fiducial"() -> (w208:bool)
            n159 = local read "Spot Name"() -> (w205:string)
            n160 = local read "MetaDataFile"() -> (w214:path)
            n161 = local read "OtherRelatedDataFiles"() -> (w204:T4)
            n162 = local write "Press to goto final Screen"(FALSE ("Press to goto final Screen")) -> ()
            n163 = local read "Z-Position"() -> (w211:dbl)
            n164 = local read "X-Position"() -> (w212:dbl)
            n165 = local read "Y-Position"() -> (w213:dbl)
            n166 = local read "MetaDataAvailable"() -> (w207:bool)
            n167 = local read "Notes:"() -> (w206:string)
            n168 = node(w210) -> (w209:dbl[unit])
            n169 = Bundle By Name(cluster=T2 {"MetaDataFile"=path "", "X"=nan, "Y"=nan, "Group"=0, "Z"=0.0, "Rotation"=0.0, "Fiducial"=FALSE, "Magnification"=0.0, "Working_Distance"=0.0, "Notes"="", "Location Name/ID"="", "OtherRelatedDataFiles"=[], "Available"=FALSE} ("Output of Spot information"), "MetaDataFile"=w214, "X"=w212, "Y"=w213, "Group"=w202, "Z"=w211, "Rotation"=w209, "Fiducial"=w208, "Magnification"=w203, "Working_Distance"=w203, "Notes"=w206, "Location Name/ID"=w205, "OtherRelatedDataFiles"=w204, "Available"=w207) -> (w216:T2)
            n170 = local write "Output of Spot information"(w216) -> ()
          }
          event "Go Back to Correct": Value Change {
            n171 = event-data() -> ()  [unwired: 1 in, 5 out]
            n172 = local write "Go Back to Correct"(FALSE ("Go Back to Correct")) -> ()
            n173 = local write "Tab Control"(T3."Name and Postions" ("Tab Control")) -> ()
          }
          event "Notes:": Value Change {
            n174 = event-data() -> ("NewVal"=w221:string)  [unwired: 1 in, 4 out]
            n175 = local read "Output of Spot information"() -> (w222:T2)
            n176 = Bundle By Name(cluster=w222, "Notes"=w221) -> (w223:T2)
            n177 = local write "Output of Spot information"(w223) -> ()
          }
        }
      }
    }
  }
  n178 = local write "MetaDataAvailable"(FALSE ("MetaDataAvailable")) -> ()
